vi "SENS_FOM_RNUM.vi"(0 "VISA IN":refnum<visa-resource-name>, 1 "Range Name":string, 5 "error in":errorcluster, 7 "Channel":i32) -> (14 "VISA Out":refnum<visa-resource-name>, 16 "Data":dbl, 19 "error out":errorcluster)   [LabVIEW 2018, in "PNA-X.lvlib"]
doc: "SENSe<cnum>:FOM:RNUM? <string> \n1737\n\n(Read-only) Returns the number of a specified range name. \nThe FOM range items are typically numbered as follows: \nPrimary 1. \nSource 2. \nReceivers 3. \nSource2 (if present) 4. \nParameters \n<cnum> Any existing channel number; if unspecified, value is set to 1. \n<string> Range name for which a number is being queried. Case insensitive. Use \nSENSe:FOM:CAT? to see a list of available range names. \nExamples SENS:FOM:RNUM? \"receivers\" \nsense2:fom:rnum? \"Source2\" \nReturn Type Numeric \nDefault Not Applicable"
uses:
  PNA-X.lvlib
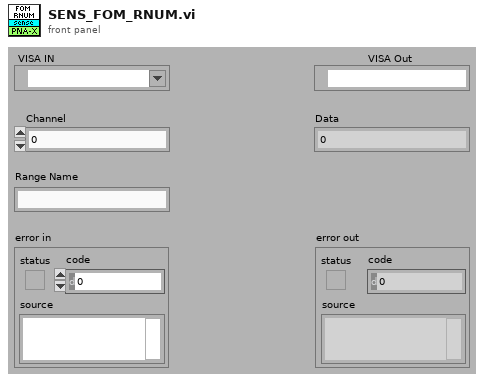
[diagram p1: front panel]
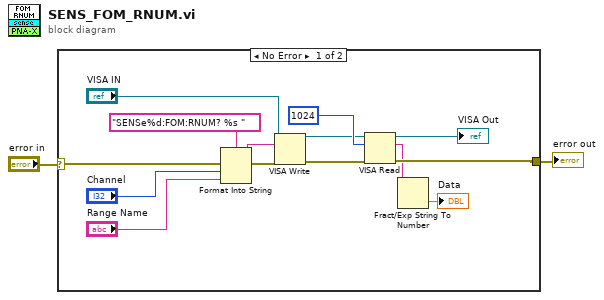
[diagram p0: block diagram]
diagram:
  n1 = case shown="No Error" "error in" {
    selector: "error in" -> [w16 w17]
    tunnel: [w7 w17] -> w1
    frame No Error {
      n2 = Format Into String(format string="SENSe%d:FOM:RNUM? %s " ("Cmdline"), error in=w16, "Channel", "Range Name") -> (resulting string=w14:string, error out=w15:errorcluster)  [unwired: 1 in]
      n3 = VISA Write(VISA resource name="VISA IN", write buffer=w14, error in (no error)=w15) -> (VISA resource name out=w9:refnum<visa-resource-name>, error out=w11:errorcluster)  [unwired: 1 out]
      n4 = VISA Read(VISA resource name=w9, byte count=1024, error in (no error)=w11) -> (VISA resource name out=→"VISA Out":refnum<visa-resource-name>, read buffer=w4:string, error out=w7:errorcluster)  [unwired: 1 out]
      n5 = Fract/Exp String To Number(string=w4) -> (number=→"Data":dbl)  [unwired: 3 in, 1 out]
    }
    frame Error {
    }
  }
  "error out" <- w1
